vi "Engine In - Sensor - CAC Outlet Pressure.vi"(10 "Loop Freq (Hz)":sgl, 11 "CAC Outlet Pressure [V]":sgl) -> (3 "CAC Outlet Pressure [kPa]":sgl)   [LabVIEW 2015, in "ECS-RT.lvlib"]
uses:
  ECS-RT.lvlib
  <vilib>/ptbypt/NI_PtbyPt.lvlib
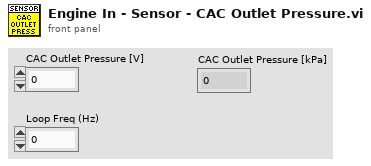
[diagram p1: front panel]
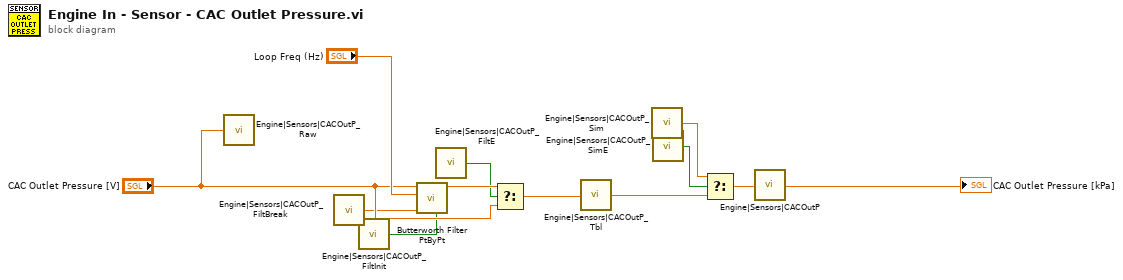
[diagram p0: block diagram]
diagram:
  n1 = call "Engine|Sensors|CACOutP_Raw"("Value"="CAC Outlet Pressure [V]") -> ()
  n2 = call "Engine|Sensors|CACOutP_FiltBreak"() -> ("Value"=w4:sgl)
  n3 = call "Engine|Sensors|CACOutP_FiltInit"() -> ("Value"=w7:bool)
  n4 = call <vilib>:"Butterworth Filter PtByPt.vi"("initialize"=w7, "low cutoff freq: fl"=w4, "sampling freq: fs"="Loop Freq (Hz)", "x"="CAC Outlet Pressure [V]") -> ("Filtered x"=w6:dbl)  [unwired: 5 in, 1 out]
  n5 = call "Engine|Sensors|CACOutP_FiltE"() -> ("Value"=w3:bool)
  n6 = Select(t=w6, s=w3, f="CAC Outlet Pressure [V]") -> (s? t:f=w5:dbl)
  n7 = call "Engine|Sensors|CACOutP_Tbl"("X Index"=w5) -> ("Y"=w2:sgl)
  n8 = call "Engine|Sensors|CACOutP_Sim"() -> ("Value"=w8:sgl)
  n9 = call "Engine|Sensors|CACOutP_SimE"() -> ("Value"=w1:bool)
  n10 = Select(t=w8, s=w1, f=w2) -> (s? t:f=w10:sgl)
  "CAC Outlet Pressure [kPa]" <- w10
  n11 = call "Engine|Sensors|CACOutP"("Value"=w10) -> ()
